vi "sc5511a_list_mode_config.vi"(0 "deviceHandle":u32 format="%.0x", 2 "List Mode Config":T1 {"Trigger Out On Cycle" items=["Trigger On Step", "Trigger On Cycle"]; "Trigger Output Enable" items=["Trigger Out Disable", "Trigger Out Enable"]; "Return to Start" items=["Stop at End", "Return to Start"]; "HW Trigger Mode" items=["Start/Stop", "Step"]; "Trigger Source" items=["Software", "Hardware"]; "Shape" items=["Sawtooth", "Triangle"]; "Direction" items=["Low to High", "High to Low"]; "Sweep / List" items=["List", "Sweep (start/stop/step)"]}, 5 "error in":errorcluster) -> (14 "deviceHandle":u32 format="%.0x", 19 "error out":errorcluster)   [LabVIEW 2010]
uses:
  sc5511a_rs232.dll
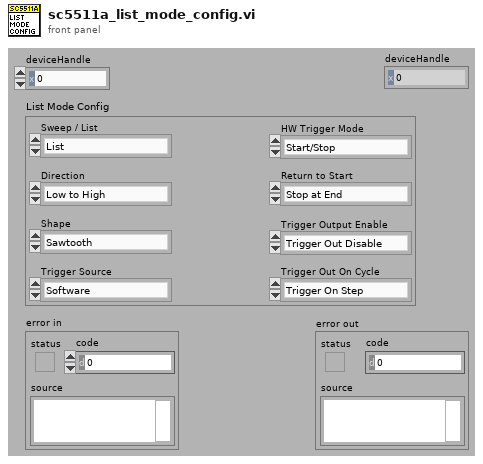
[diagram p1: front panel]
types:
  T1 = cluster{"Sweep / List":u8, "Direction":u8, "Shape":u8, "Trigger Source":u8, "HW Trigger Mode":u8, "Return to Start":u8, "Trigger Output Enable":u8, "Trigger Out On Cycle":u8}
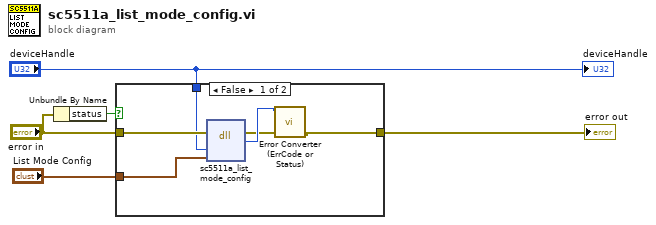
[diagram p0: block diagram]
diagram:
  n1 = Unbundle By Name("error in") -> ("status"=w5:bool)
  n2 = case shown="False" w5 {
    tunnel: "error in" -> [w11 w12]
    tunnel: [w9 w12] -> w2
    tunnel: "deviceHandle" -> [w7 _]
    tunnel: "List Mode Config" -> [w6 _]
    frame False {
      n3 = dll-call lib="sc5511a_rs232.dll" fn="sc5511a_list_mode_config"(error in=w11, "deviceHandle"=w7, "mode_config_t"=w6) -> (error out=w8:errorcluster, "return type"=w10:i32)  [unwired: 4 in, 1 out]
      n4 = call "Error Converter (ErrCode or Status).vi"("error in (no error)"=w8, "error code"=w10) -> ("error out"=w9:errorcluster)  [unwired: 9 in]
    }
    frame True {
    }
  }
  "error out" <- w2
  "deviceHandle" <- "deviceHandle"
